vi "Process.vi"(8 "error in":errorcluster, 11 "Instrument.Example":refnum<class "Instrument.OxfordVRM.lvclass">) -> (0 "error out":errorcluster, 3 "Instrument.Example out":refnum<class "Instrument.OxfordVRM.lvclass">)   [LabVIEW 2016, in "Instrument.OxfordVRM.lvclass"]
doc: "---------------------------------------------------------------\nJKI State Machine Objects™\nhttp://jki.net/state-machine-objects/\nCopyright (C) 2005-2015, JKI <info@jki.net>\nALL RIGHTS RESERVED"
uses:
  Instrument.OxfordVRM.lvclass
  C:/Program Files (x86)/National Instruments/LabVIEW 2016/vi.lib/JKI/JKI SMO/SMO/SMO.lvclass
  <vilib>/JKI/JKI SMO/SMO/Typedefs/Parent Call--Enum.ctl
  <instrlib>/Mercury iXX/Public/Libraries/Magnet/Controls/Switch Heater.ctl
  <userlib>/LevyLab/Levylab Instruments/Instrument Types/Cryostat/Instrument.Cryostat.lvclass
  <vilib>/JKI/JKI SMO/SMO/SMO.lvclass
  <instrlib>/Mercury iXX/Public/Libraries/Magnet.lvlib
panel:
  out "State":string
  out "timer":u32
  # "For instructions on how to use the JKI State Machine Objects, examples and video tutorials, visit:\nhttp://jki.net/state-machine-objects/\n\nJKI State Machine Objects™\nhttp://jki.net/state-machine-objects/\nCopyright (C) 2005-2015, JKI <info@jki.net>\nALL RIGHTS RESERVED"
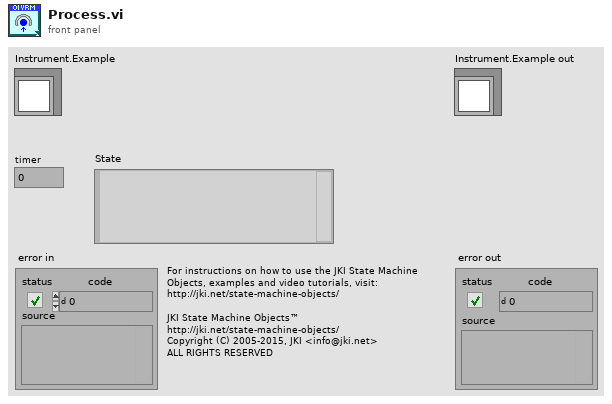
[diagram p1: front panel]
types:
  T1 = typedef "SMO.lvclass/Parent Call--Enum.ctl" = enum16{"Allows parent to run", "Does not request parent to run"}
  T2 = enum32{"invalid app kind", "Development System", "Run Time System", "Student Edition", "Embedded LabVIEW", "Evaluation", "Custom"}
  T3 = enum32{"Invalid", "Standard", "Closed", "Hidden", "Minimized", "Maximized"}
  T4 = enum32{"Bad", "Idle", "Run top level", "Running"}
  T5 = typedef "Mercury iXX.lvlib/Magnet.lvlib/Switch Heater.ctl" = string
  T6 = cluster{"Core":cluster{"Current VI Reference":refnum<vi>, "Close Panel on Exit?":bool, "error":errorcluster}, "Self Reference":refnum<class "Instrument.OxfordVRM.lvclass">, "Field (T)":dbl, "Field Rate (T/min)":dbl, "persistent":bool, "Running Step":i32, "sequence":string[]}
  T7 = cluster{"Current VI Reference":refnum<vi>, "Close Panel on Exit?":bool, "error":errorcluster}
  T8 = typedef "SMO.lvclass/Protected Events.ctl" = cluster{"StopProcesses":refnum<user-event>, "AbortProcesses":refnum<user-event>, "Config Changed":refnum<user-event>, "Dependency":refnum<user-event>}
  T9 = typedef "Instrument.OxfordVRM.lvclass/PrivateEvents--Cluster.ctl" = cluster{"SequenceSetMagnetField":refnum<user-event>, "AbortSequence":refnum<user-event>}
  T10 = cluster{"Holding":bool, "Ramp to Setpoint":bool, "Ramp to Zero":bool, "Clamp":bool}
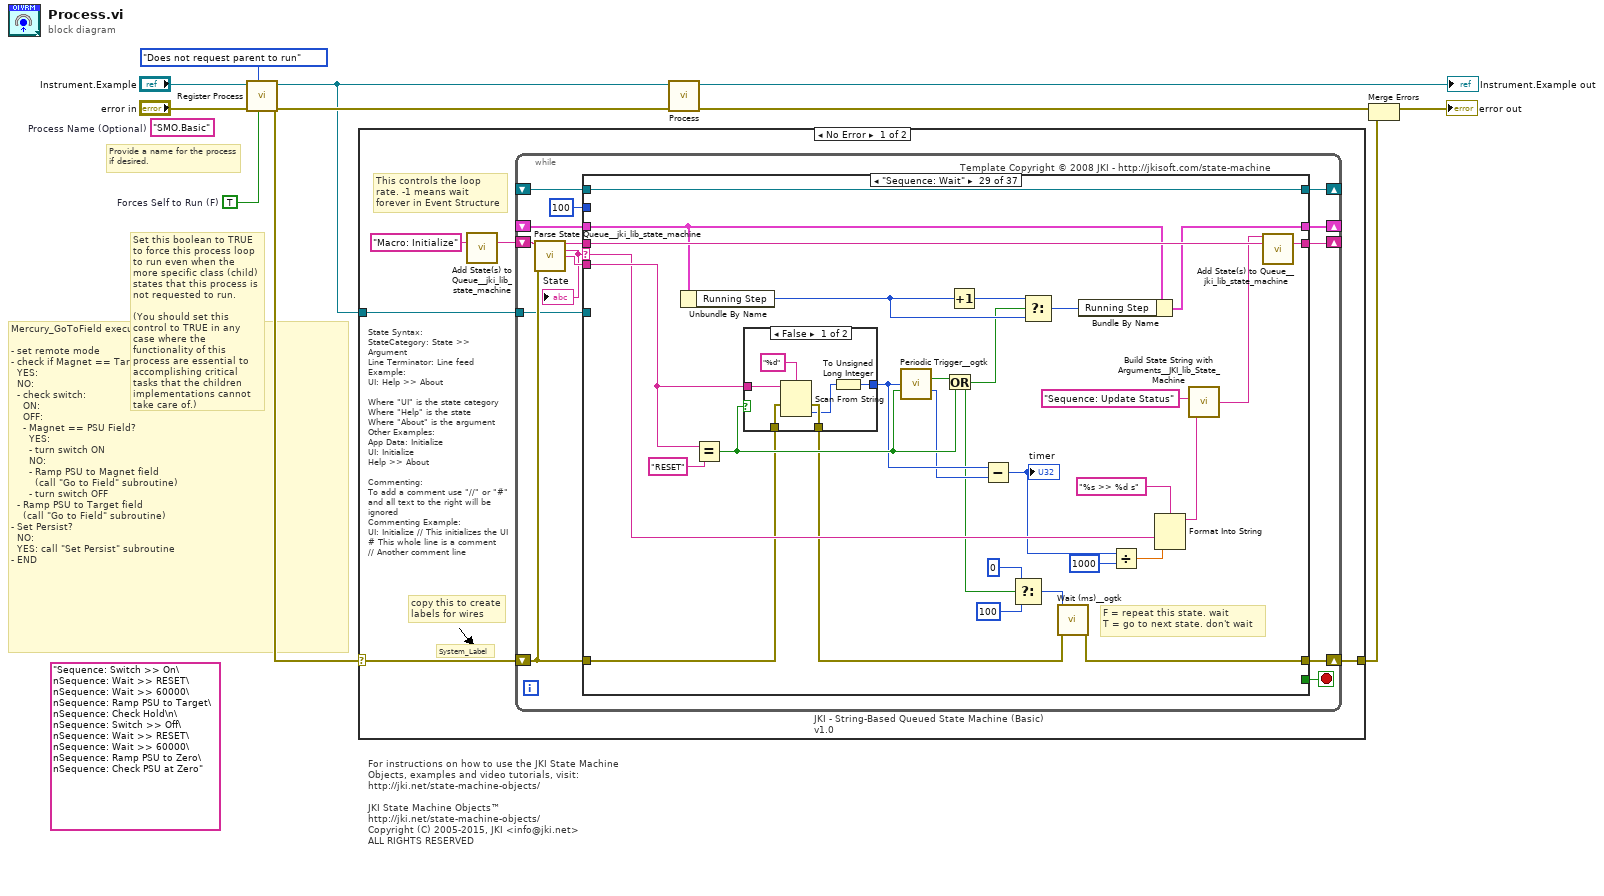
[diagram p0: block diagram]
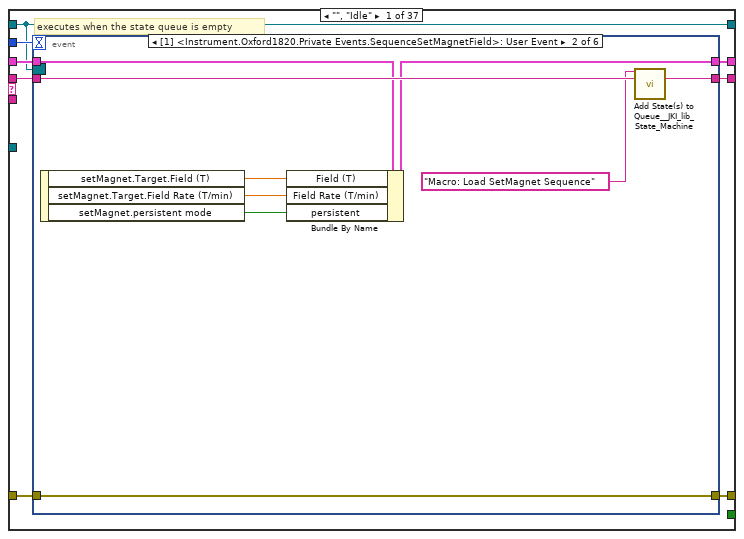
[diagram p2: hidden frame]
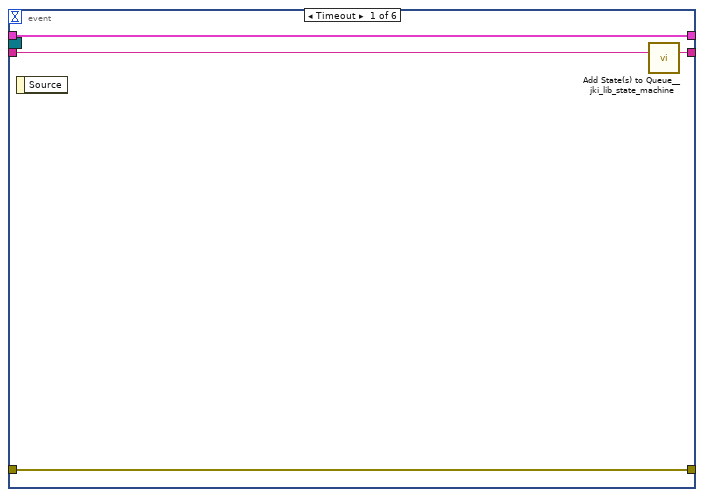
[diagram p3: hidden frame]
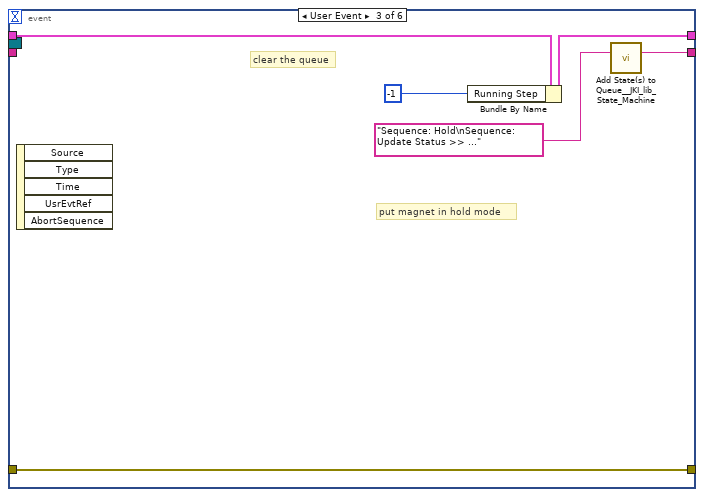
[diagram p4: hidden frame]
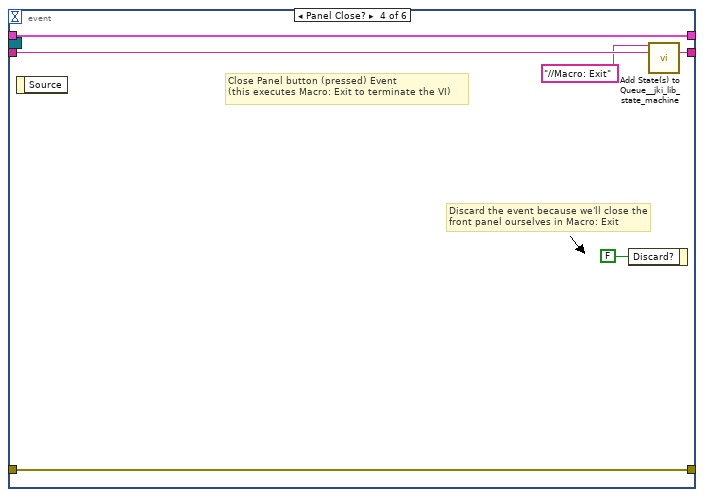
[diagram p5: hidden frame]
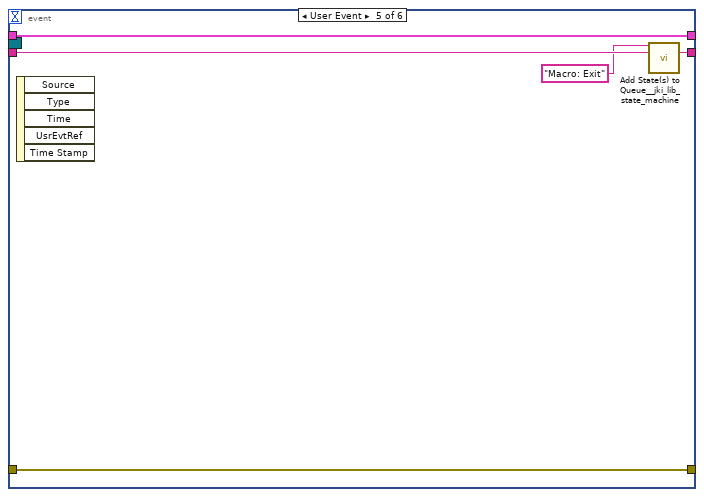
[diagram p6: hidden frame]
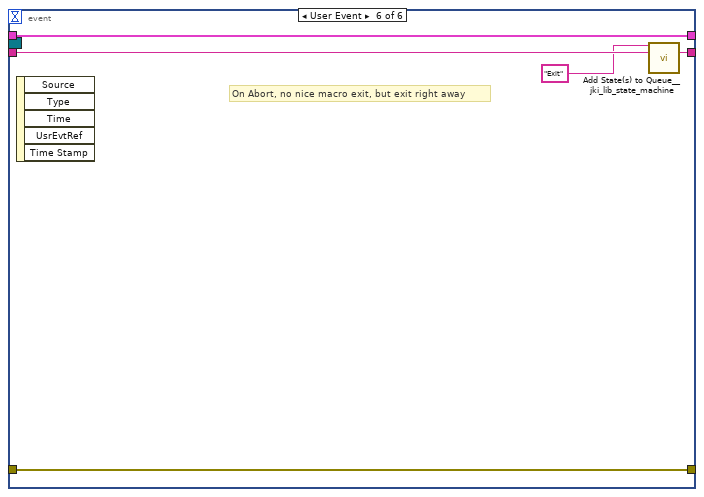
[diagram p7: hidden frame]
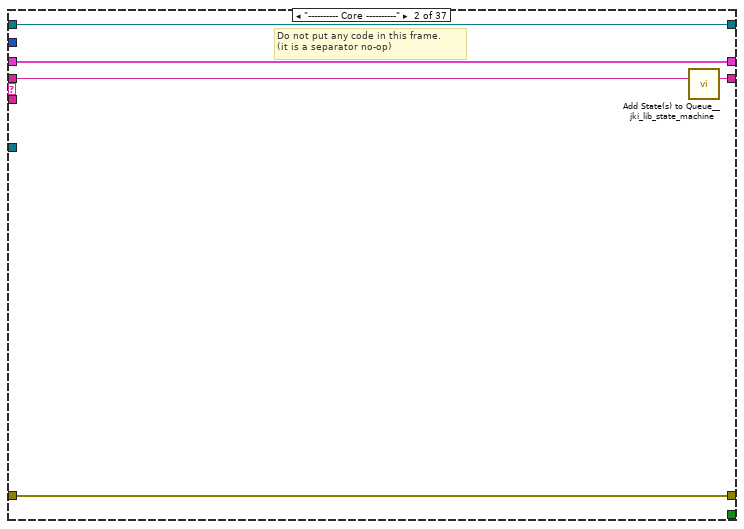
[diagram p8: hidden frame]
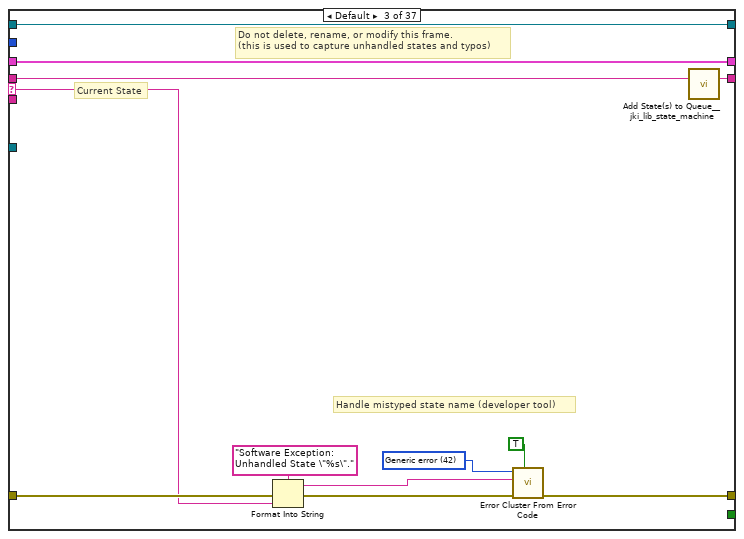
[diagram p9: hidden frame]
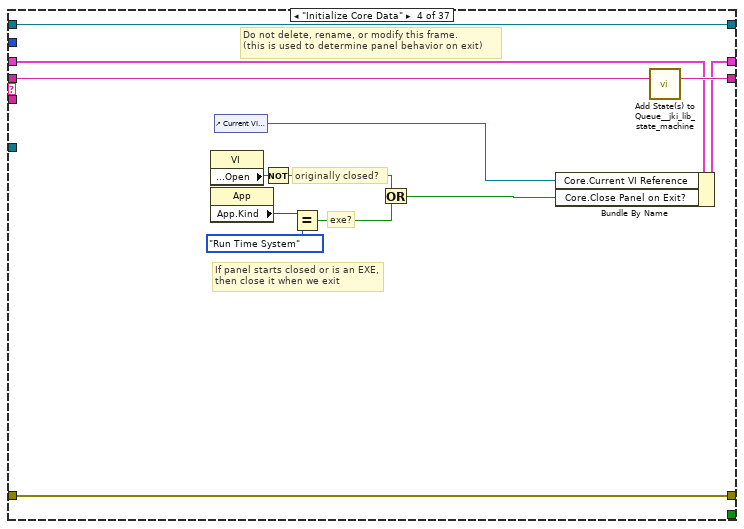
[diagram p10: hidden frame]
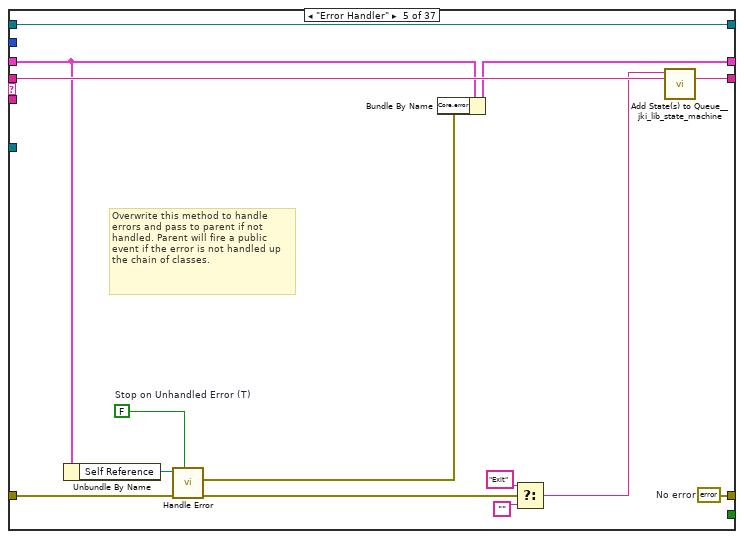
[diagram p11: hidden frame]
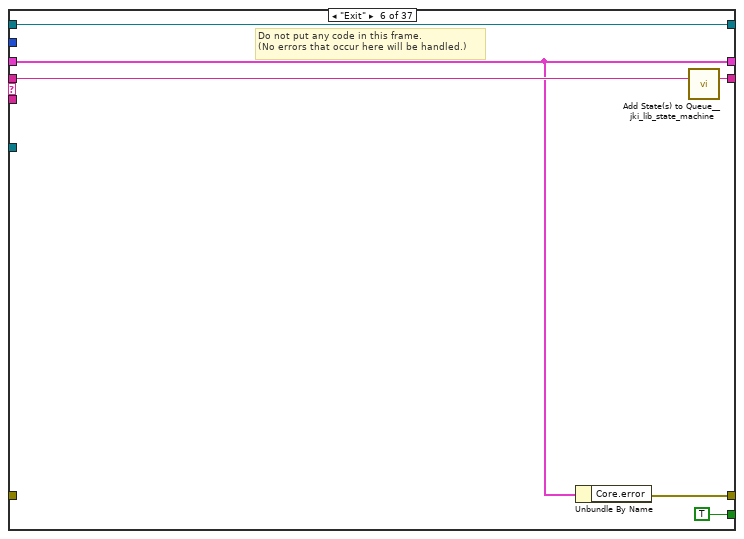
[diagram p12: hidden frame]
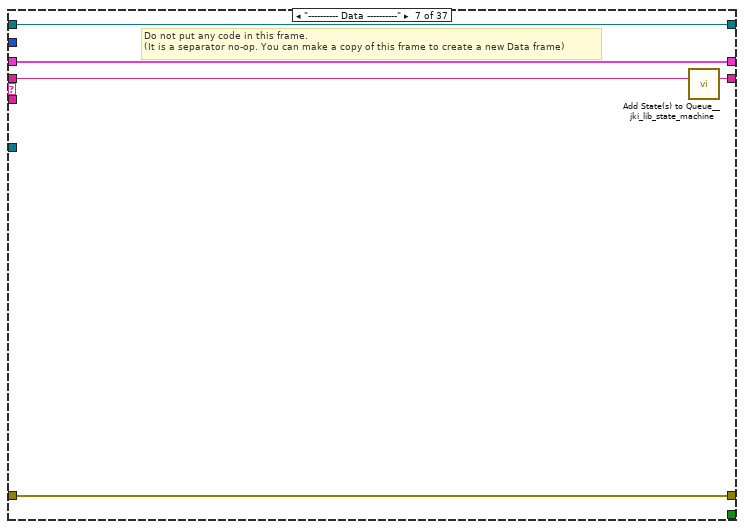
[diagram p13: hidden frame]
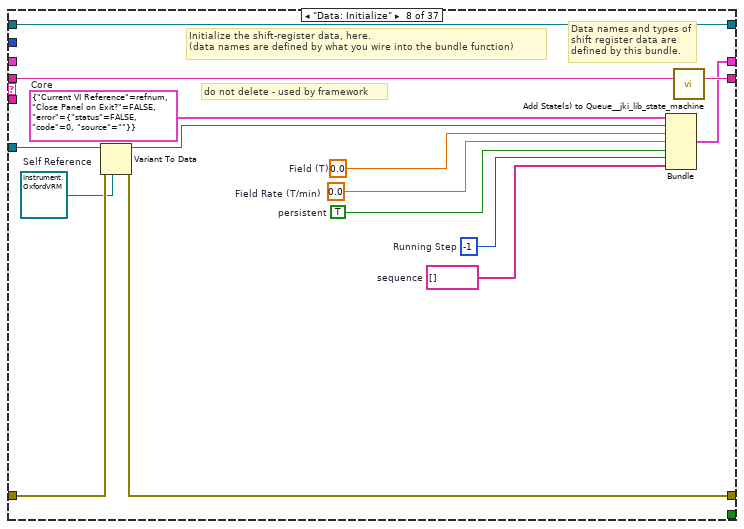
[diagram p14: hidden frame]
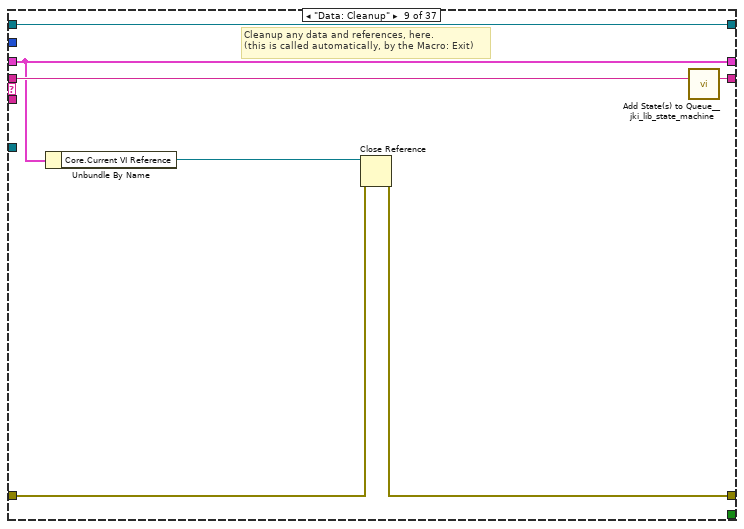
[diagram p15: hidden frame]
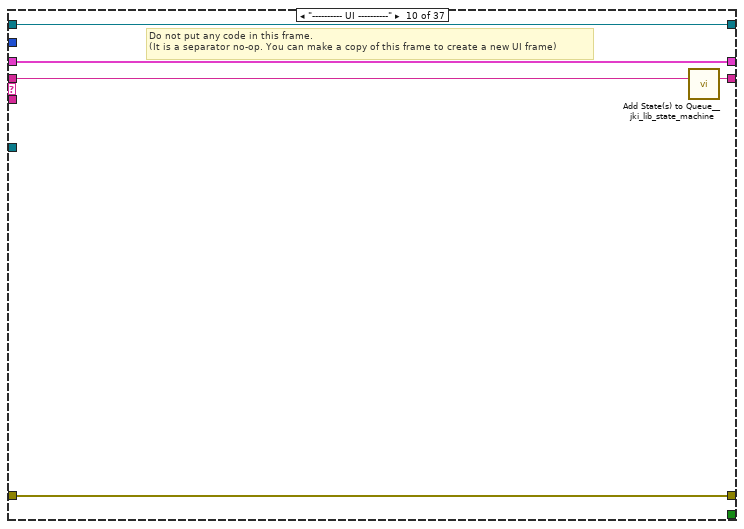
[diagram p16: hidden frame]
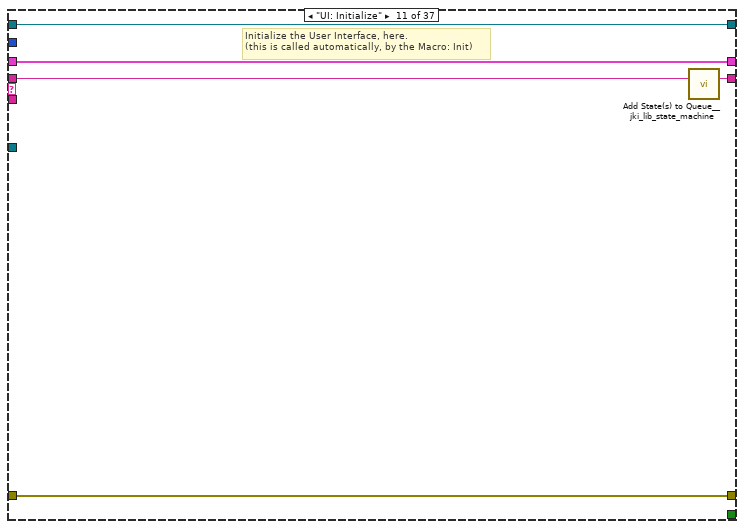
[diagram p17: hidden frame]
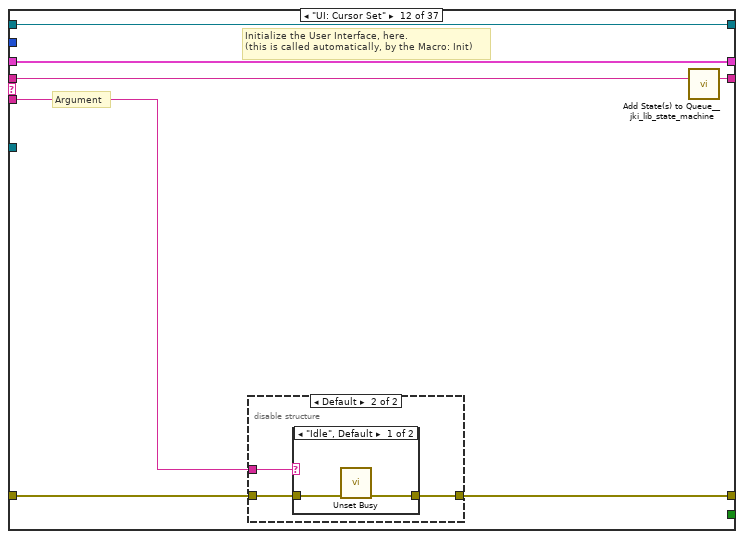
[diagram p18: hidden frame]
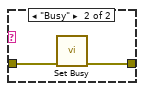
[diagram p20: hidden frame]
diagram:
  (unwired) "Sequence: Switch >> On\nSequence: Wait >> RESET\nSequence: Wait >> 60000\nSequence: Ramp PSU to Target\nSequence: Check Hold\n\nSequence: Switch >> Off\nSequence: Wait >> RESET\nSequence: Wait >> 60000\nSequence: Ramp PSU to Zero\nSequence: Check PSU at Zero" ("State(s) in Front (\"\")")
  w1 = TRUE  # Forces Self to Run (F)
  (unwired) "SMO.Basic"  # Process Name (Optional)
  # "Mercury_GoToField executes the following states:\n\n- set remote mode\n- check if Magnet == Target.\n  YES:\n  NO:\n  - check switch:\n    ON:\n    OFF:\n    - Magnet == PSU Field?\n      YES:\n      - turn switch ON\n      NO:\n      - Ramp PSU to Magnet field\n        (call \"Go to Field\" subroutine)\n      - turn switch OFF\n  - Ramp PSU to Target field\n    (call \"Go to Field\" subroutine)\n- Set Persist?\n  NO:\n  YES: call \"Set Persist\" subroutine\n- END"
  # "Provide a name for the process\nif desired."
  # "Set this boolean to TRUE to force this process loop to run even when the more specific class (child) states that this process is not requested to run.\n\n(You should set this control to TRUE in any case where the functionality of this process are essential to accomplishing critical tasks that the children implementations cannot take care of.)"
  # "For instructions on how to use the JKI State Machine Objects, examples and video tutorials, visit:\nhttp://jki.net/state-machine-objects/\n\nJKI State Machine Objects™\nhttp://jki.net/state-machine-objects/\nCopyright (C) 2005-2015, JKI <info@jki.net>\nALL RIGHTS RESERVED"
  n1 = call <vilib>:"Register Process.vi"("Forces Self to Run (F)"=w1, "Parent Call"=Parent_Call--Enum."Does not request parent to run", "error in (no error)"="error in", "SMO"="Instrument.Example") -> ("error out"=w7:errorcluster, "SMO out"=w6:refnum<class "Instrument.OxfordVRM.lvclass">)  [unwired: 6 in]
  n2 = case shown="No Error" w7 {
    selector: w7 -> [w12 w608]
    tunnel: w6 -> [w13 _]
    tunnel: [w11 w608] -> w3
    frame No Error {
      # "State Syntax:\nStateCategory: State >> Argument\nLine Terminator: Line feed\nExample:\nUI: Help >> About\n\nWhere \"UI\" is the state category\nWhere \"Help\" is the state\nWhere \"About\" is the argument\nOther Examples:\nApp Data: Initialize\nUI: Initialize\nHelp >> About\n\nCommenting:\nTo add a comment use \"//\" or \"#\" and all text to the right will be ignored\nCommenting Example:\nUI: Initialize // This initializes the UI\n# This whole line is a comment\n// Another comment line"
      # "copy this to create labels for wires"
      # "This controls the loop rate. -1 means wait forever in Event Structure"
      # "System_Label"
      n3 = call <vilib>:"Add State(s) to Queue__jki_lib_state_machine.vi"("State(s) in (\"\")"="Macro: Initialize") -> ("States Out"=w15:string)  [unwired: 14 in]
      n4 = while "JKI - String-Based Queued State Machine (Basic) v1.0" {
        shift-right: [w23] -> _
        shift-left: _ -> [w22]
        shift-right: [w26] -> w11
        shift-left: w12 -> [w20]
        shift-right: [w25] -> _
        shift-left: w15 -> [w27]
        tunnel: w13 -> [w19]
        shift-right: [w18] -> _
        shift-left: _ -> [w17]
        stop <- w24 stop-if-true
        # "Template Copyright © 2008 JKI - http://jkisoft.com/state-machine"
        n5 = call <vilib>:"Parse State Queue__jki_lib_state_machine.vi"("State Queue"=w27, "Error In (no error)"=w20) -> ("Remaining States"=w29:string, "Current State"=w16:string, "Arguments"=w28:string)  [unwired: 11 in]
        "State" <- w16
        n6 = case shown="\"Sequence: Wait\"" w16 {
          selector: w16 -> [_ _ w79 _ _ _ _ _ _ _ _ _ _ _ _ _ _ _ _ _ _ _ _ _ _ _ w363 w379 w407 w431 w460 w492 w509 w529 w549 w568 w598]
          tunnel: w29 -> [w37 w77 w83 w102 w116 w122 w127 w142 w149 w154 w159 w166 w182 w214 w235 w249 w266 _ w297 w308 w313 w326 w332 w341 w348 w358 w372 w389 w420 w447 w477 w500 w519 w539 w559 w580 w607]
          tunnel: w28 -> [_ _ _ _ _ _ _ _ _ _ _ w160 w176 _ _ _ _ _ _ _ _ _ _ _ _ w350 _ w378 w408 _ _ _ _ _ _ _ _]
          tunnel: w22 -> [w35 w74 w81 w93 w110 w118 w124 _ w144 w151 w157 w164 w178 w211 w232 w240 w254 w274 w294 w305 w310 w324 w330 w335 w344 w355 w369 w384 w393 w440 w473 w497 w512 w532 w552 w577 w604]
          tunnel: [w34 w75 w85 w99 w111 w117 w125 w138 w145 w152 w156 w161 w179 w212 w221 w247 w264 w270 w295 w299 w311 w319 w328 w338 w345 w351 w366 w381 w397 w434 w469 w488 w501 w521 w541 w560 w597] -> w26
          tunnel: w20 -> [w33 w75 w84 w99 w112 _ w125 w139 w146 w152 w156 w162 w180 w212 w222 w247 w264 w271 w295 w300 w311 w320 w328 w338 w345 w352 w361 w374 w396 w429 w458 w489 _ w520 w540 w562 w592]
          tunnel: [w36 w76 w82 w101 w115 w121 w126 w141 w148 w153 w158 w165 w181 w213 w234 w248 w265 w285 w296 w307 w312 w325 w331 w340 w347 w357 w371 w388 w419 w446 w476 w499 w518 w538 w558 w579 w606] -> w25
          tunnel: [_ _ _ _ _ TRUE _ _ _ _ _ _ _ _ _ _ _ _ _ _ _ _ _ _ _ _ _ _ _ _ _ _ _ _ _ _ _] -> w24
          tunnel: [w32 w74 w81 w100 w109 w118 w124 w140 w144 w151 w157 w164 w178 w211 w232 w240 w262 w275 w294 w305 w310 w324 w330 w334 w343 w354 w368 w383 w417 w439 w472 w496 w511 w531 w551 w576 w603] -> w23
          tunnel: 100 ("Timeout") -> [w31 _ _ _ _ _ _ _ _ _ _ _ _ _ _ _ _ _ _ _ _ _ _ _ _ _ _ _ _ _ _ _ _ _ _ _ _]
          tunnel: w19 -> [_ _ _ _ _ _ _ w136 _ _ _ _ _ _ w223 _ _ _ _ _ _ _ _ _ _ _ _ _ _ _ _ _ _ _ _ _ _]
          tunnel: [w30 w73 w78 w90 w114 w119 w123 w134 w143 w150 w155 w163 w175 w210 w233 w241 w263 w284 w293 w306 w309 w323 w329 w339 w346 w356 w370 w387 w418 w445 w475 w498 w517 w537 w557 w578 w605] -> w18
          tunnel: w17 -> [w30 w73 w78 w90 w114 w119 w123 w134 w143 w150 w155 w163 w175 w210 w233 w241 w263 w284 w293 w306 w309 _ w329 w339 w346 w356 w370 w387 w418 w445 w475 w498 w517 w537 w557 w578 w605]
          frame "", "Idle" {
            # "executes when the state queue is empty"
            n7 = event shown="[1] <Instrument.Oxford1820.Private Events.SequenceSetMagnetField>: User Event" {
              selector: w30 -> [_ _ _ _ _ _]
              dyn-events: _ -> [_ _ _ _ _ _]
              timeout: w31 -> [_ _ _ _ _ _]
              tunnel: w37 -> [w41 w48 _ w62 w67 w72]
              tunnel: [w40 w49 w55 w61 w66 w71] -> w36
              tunnel: w35 -> [w38 w44 w53 w59 w64 w69]
              tunnel: [w39 w50 w56 w60 w65 w70] -> w34
              tunnel: w33 -> [w39 w50 w56 w60 w65 w70]
              tunnel: [w38 w43 w52 w59 w64 w69] -> w32
              event Timeout {
                n8 = event-data() -> ()  [unwired: 1 in, 1 out]
                n9 = call <vilib>:"Add State(s) to Queue__jki_lib_state_machine.vi"("State(s) in (\"\")"=w41) -> ("States Out"=w40:string)  [unwired: 14 in]
              }
              event User Event {
                n10 = event-data() -> ("setMagnet.Target.Field (T)"=w47:dbl, "setMagnet.Target.Field Rate (T/min)"=w46:dbl, "setMagnet.persistent mode"=w45:bool)  [unwired: 1 in]
                n11 = Bundle By Name(cluster=w44, "Field (T)"=w47, "Field Rate (T/min)"=w46, "persistent"=w45) -> (w43:T6)
                n12 = call <vilib>:"Add State(s) to Queue__JKI_lib_State_Machine.vi"("State(s) in Front (\"\")"="Macro: Load SetMagnet Sequence" ("State(s) at Back (\"\")"), "State(s) in (\"\")"=w48) -> ("States Out"=w49:string)  [unwired: 13 in]
              }
              event User Event {
                # "put magnet in hold mode"
                # "clear the queue"
                n13 = event-data() -> ()  [unwired: 1 in, 5 out]
                n14 = Bundle By Name(cluster=w53, "Running Step"=-1) -> (w52:T6)
                n15 = call <vilib>:"Add State(s) to Queue__JKI_lib_State_Machine.vi"("State(s) in (\"\")"="Sequence: Hold\nSequence: Update Status >> ..." ("State(s) at Back (\"\")")) -> ("States Out"=w55:string)  [unwired: 14 in]
              }
              event Panel Close? {
                # "Discard the event because we'll close the front panel ourselves in Macro: Exit"
                # "Close Panel button (pressed) Event\n(this executes Macro: Exit to terminate the VI)"
                n16 = event-data() -> ()  [unwired: 1 in, 1 out]
                n17 = event-data("Discard?"=FALSE) -> ()  [unwired: 1 in, 1 out]
                n18 = call <vilib>:"Add State(s) to Queue__jki_lib_state_machine.vi"("State(s) in Front (\"\")"="//Macro: Exit", "State(s) in (\"\")"=w62) -> ("States Out"=w61:string)  [unwired: 13 in]
              }
              event User Event {
                n19 = event-data() -> ()  [unwired: 1 in, 5 out]
                n20 = call <vilib>:"Add State(s) to Queue__jki_lib_state_machine.vi"("State(s) in Front (\"\")"="Macro: Exit", "State(s) in (\"\")"=w67) -> ("States Out"=w66:string)  [unwired: 13 in]
              }
              event User Event {
                # "On Abort, no nice macro exit, but exit right away"
                n21 = event-data() -> ()  [unwired: 1 in, 5 out]
                n22 = call <vilib>:"Add State(s) to Queue__jki_lib_state_machine.vi"("State(s) in Front (\"\")"="Exit", "State(s) in (\"\")"=w72) -> ("States Out"=w71:string)  [unwired: 13 in]
              }
            }
          }
          frame "---------- Core ----------" {
            # "Do not put any code in this frame.\n(it is a separator no-op)"
            n23 = call <vilib>:"Add State(s) to Queue__jki_lib_state_machine.vi"("State(s) in (\"\")"=w77) -> ("States Out"=w76:string)  [unwired: 14 in]
          }
          frame Default {
            w88 = 42 items=["No error", "Argument error", "Memory is full", "Out of zone", "End of file", "File already open", "Generic file I/O error", "File not found", "File permission error", "Disk is full", "Duplicate path", "Too many files open", "System feature not enabled", "Resource file not found", "Cannot add resource", "Resource not found", "Image not found", "Image memory error", "Pen does not exist", "Config type invalid", "Config token not found", "Config parse error", "Config memory error", "Bad external code format", "Bad external code offset", "External code not present", "Null window", "Destroy window error", "Null menu", "Print aborted", "Bad print record", "Print driver error", "Windows error during printing", "Memory error during printing", "Print dialog error", "Generic print error", "Invalid device refnum", "Device not found", "Device parameter error", "Device unit error", "Cannot open device", "Device call aborted", "Generic error", "Cancelled by user", "Object ID too low", "Object ID too high", "Object not in heap", "Unknown heap", "Unknown object (invalid DefProc)", "Unknown object (DefProc not in table)", "Message out of range", "Invalid (null) method", "Unknown message", "Manager call not supported", "Bad address", "Network operation in progress", "Network operation timed out", "Connection is busy", "Network attribute not supported", "Network error", "Address in use", "System out of memory", "Connection aborted", "Connection refused", "Not connected", "Already connected", "Connection closed", "Initialization error (interapplication manager)", "Bad occurrence", "Wait on unbound occurrence handler", "Occurrence queue overflow", "Datalog type conflict", "Unused", "Unrecognized type (interapplication manager)", "Memory corrupt", "Failed to make temporary DLL", "Old CIN version", "Drag socket not found", "Failed to load drop-object", "Failed to register OLE object", "Failed to release OLE object", "Format specifier type mismatch", "Unknown format specifier", "Too few format specifiers", "Too many format specifiers", "Scan failed", "Newer CIN version", "Error converting to variant", "Runtime menu error", "Password tampered", "Variant attribute not found", "Incompatible variant data type", "Event data is not available", "Event Store is not present", "Occurrence is not found", "Event Queue is not created", "Event info is not available", "Refnum passed is NULL", "Error retrieving Class GUID", "Error retrieving CoClass GUID", "Error retrieving TypeLib GUID.", "Bad built application magic bytes.", "Specific driver is different from the specific driver associated with the Logical Name.", "There is no session opened to the class driver.", "Max Error", "MAX - Error with config objects", "MAX - Error loading configuration", "MAX - Group not supported"]
            # "Current State"
            # "Do not delete, rename, or modify this frame.\n(this is used to capture unhandled states and typos)"
            # "Handle mistyped state name (developer tool)"
            n24 = Format Into String(format string="Software Exception: Unhandled State \"%s\"." ("message"), error in=w84, w79) -> (resulting string=w87:string, error out=w86:errorcluster)  [unwired: 1 in]
            n25 = call <vilib>:"Error Cluster From Error Code.vi"("show call chain? (False)"=TRUE, "error in (no error)"=w86, "error message (\"\")"=w87, "error code (0)"=w88) -> ("error out"=w85:errorcluster)  [unwired: 5 in]
            n26 = call <vilib>:"Add State(s) to Queue__jki_lib_state_machine.vi"("State(s) in (\"\")"=w83) -> ("States Out"=w82:string)  [unwired: 14 in]
          }
          frame "Initialize Core Data" {
            # "Do not delete, rename, or modify this frame.\n(this is used to determine panel behavior on exit)"
            # "originally closed?"
            # "exe?"
            # "If panel starts closed or is an EXE, then close it when we exit"
            n27 = property class="VI"() -> ("Front Panel.Open"=w98:bool)  [unwired: 2 in, 2 out]
            n28 = property class="App"() -> ("App.Kind"=w97:T2)  [unwired: 2 in, 2 out]
            n29 = control-ref of="Current VI Reference"() -> (w91:refnum<vi>)
            n30 = Not(x=w98) -> (.not. x?=w95:bool)
            n31 = Equal?(x=w97, y=T2."Run Time System" ("Application:Kind")) -> (x = y?=w94:bool)
            n32 = Or(x=w95, y=w94) -> (x .or. y?=w92:bool)
            n33 = Bundle By Name(cluster=w93, "Core.Current VI Reference"=w91, "Core.Close Panel on Exit?"=w92) -> (w100:T6)
            n34 = call <vilib>:"Add State(s) to Queue__jki_lib_state_machine.vi"("State(s) in (\"\")"=w102) -> ("States Out"=w101:string)  [unwired: 14 in]
          }
          frame "Error Handler" {
            w103 = FALSE  # Stop on Unhandled Error (T)
            w111 = errorcluster {"status"=FALSE, "code"=0, "source"=""}  # No error
            # "Overwrite this method to handle errors and pass to parent if not handled. Parent will fire a public event if the error is not handled up the chain of classes."
            n35 = Unbundle By Name(w110) -> ("Self Reference"=w113:refnum<class "Instrument.OxfordVRM.lvclass">)
            n36 = call-dynamic "Handle Error.vi"("Stop on Unhandled Error (T)"=w103, "error in"=w112, "Instrument"=w113) -> ("handling error"=w104:errorcluster, "Unhandled error"=w107:errorcluster)  [unwired: 6 in, 1 out]
            n37 = Bundle By Name(cluster=w110, "Core.error"=w107) -> (w109:T6)
            n38 = Select(t="Exit", s=w104, f="") -> (s? t:f=w108:string)
            n39 = call <vilib>:"Add State(s) to Queue__jki_lib_state_machine.vi"("State(s) in Front (\"\")"=w108, "State(s) in (\"\")"=w116) -> ("States Out"=w115:string)  [unwired: 13 in]
          }
          frame "Exit" {
            # "Do not put any code in this frame.\n(No errors that occur here will be handled.)"
            n40 = Unbundle By Name(w118) -> ("Core.error"=w117:errorcluster)
            n41 = call <vilib>:"Add State(s) to Queue__jki_lib_state_machine.vi"("State(s) in (\"\")"=w122) -> ("States Out"=w121:string)  [unwired: 14 in]
          }
          frame "---------- Data ----------" {
            # "Do not put any code in this frame.\n(It is a separator no-op. You can make a copy of this frame to create a new Data frame)"
            n42 = call <vilib>:"Add State(s) to Queue__jki_lib_state_machine.vi"("State(s) in (\"\")"=w127) -> ("States Out"=w126:string)  [unwired: 14 in]
          }
          frame "Data: Initialize" {
            w128 = string[] []  # sequence
            w129 = -1  # Running Step
            w130 = TRUE  # persistent
            w131 = 0.0  # Field Rate (T/min)
            w132 = 0.0  # Field (T)
            w133 = T7 {"Current VI Reference"=refnum, "Close Panel on Exit?"=FALSE, "error"={"status"=FALSE, "code"=0, "source"=""}}  # Core
            w137 = refnum<class "Instrument.OxfordVRM.lvclass"> refnum  # Self Reference
            # "do not delete - used by framework"
            # "Data names and types of shift register data are defined by this bundle."
            # "Initialize the shift-register data, here.\n(data names are defined by what you wire into the bundle function)"
            n43 = Variant To Data(error in=w139, type=w137, Variant=w136) -> (data=w135:refnum<class "Instrument.OxfordVRM.lvclass">, error out=w138:errorcluster)
            n44 = Bundle("Core"=w133, "Self Reference"=w135, "Field (T)"=w132, "Field Rate (T/min)"=w131, "persistent"=w130, "Running Step"=w129, "sequence"=w128) -> (w140:T6)  [unwired: 1 in]
            n45 = call <vilib>:"Add State(s) to Queue__jki_lib_state_machine.vi"("State(s) in (\"\")"=w142) -> ("States Out"=w141:string)  [unwired: 14 in]
          }
          frame "Data: Cleanup" {
            # "Cleanup any data and references, here.\n(this is called automatically, by the Macro: Exit)"
            n46 = Unbundle By Name(w144) -> ("Core.Current VI Reference"=w147:refnum<vi>)
            n47 = Close Reference(reference=w147, error in (no error)=w146) -> (error out=w145:errorcluster)
            n48 = call <vilib>:"Add State(s) to Queue__jki_lib_state_machine.vi"("State(s) in (\"\")"=w149) -> ("States Out"=w148:string)  [unwired: 14 in]
          }
          frame "---------- UI ----------" {
            # "Do not put any code in this frame.\n(It is a separator no-op. You can make a copy of this frame to create a new UI frame)"
            n49 = call <vilib>:"Add State(s) to Queue__jki_lib_state_machine.vi"("State(s) in (\"\")"=w154) -> ("States Out"=w153:string)  [unwired: 14 in]
          }
          frame "UI: Initialize" {
            # "Initialize the User Interface, here.\n(this is called automatically, by the Macro: Init)"
            n50 = call <vilib>:"Add State(s) to Queue__jki_lib_state_machine.vi"("State(s) in (\"\")"=w159) -> ("States Out"=w158:string)  [unwired: 14 in]
          }
          frame "UI: Cursor Set" {
            # "Argument"
            # "Initialize the User Interface, here.\n(this is called automatically, by the Macro: Init)"
            n51 = disable-structure shown="Default" {
              disable-tunnel: w162 -> [w167 w170]
              disable-tunnel: [w167 w169] -> w161
              disable-tunnel: w160 -> [_ w168]
              frame condition #0 {
              }
              frame condition #1 (active) {
                n52 = case shown="\"Idle\", Default" w168 {
                  tunnel: w170 -> [w172 w174]
                  tunnel: [w171 w173] -> w169
                  frame "Idle", Default {
                    n53 = call <vilib>:"Unset Busy.vi"("error in (no error)"=w172) -> ("error out"=w171:errorcluster)  [unwired: 10 in]
                  }
                  frame "Busy" {
                    n54 = call <vilib>:"Set Busy.vi"("error in (no error)"=w174) -> ("error out"=w173:errorcluster)  [unwired: 9 in, 1 out]
                  }
                }
              }
            }
            n55 = call <vilib>:"Add State(s) to Queue__jki_lib_state_machine.vi"("State(s) in (\"\")"=w166) -> ("States Out"=w165:string)  [unwired: 14 in]
          }
          frame "UI: Front Panel State" {
            # "Argument"
            # "Set Front Panel Open or Closed\n(Usage: \"UI: Front Panel State >> Open|Close\")"
            n56 = Unbundle By Name(w178) -> ("Core.Current VI Reference"=w177:refnum<vi>)
            n57 = disable-structure shown="Default" {
              disable-tunnel: w180 -> [w186 w209]
              disable-tunnel: [w185 w209] -> w179
              disable-tunnel: w177 -> [w184 _]
              disable-tunnel: w176 -> [w183 _]
              frame condition #0 (active) {
                n58 = case shown="\"Close\"" w183 {
                  tunnel: w186 -> [w190 w203]
                  tunnel: [w192 w204] -> w185
                  tunnel: w184 -> [w191 w201]
                  frame "Open", Default {
                    n59 = property class="VI"(reference=w191, error in=w190) -> (reference out=w188:refnum<vi>, error out=w189:errorcluster, "FP.State"=w187:T3)
                    n60 = case shown="\"Closed\"" w187 {
                      tunnel: [w195 w198] -> w192
                      tunnel: w189 -> [w194 w198]
                      tunnel: w188 -> [w193 _]
                      frame "Closed" {
                        n61 = invoke class="VI" method="FP.Open"(reference=w193, error in=w194, "Activate"=TRUE, "State"=T3."Standard") -> (error out=w195:errorcluster)  [unwired: 1 in, 4 out]
                      }
                      frame Default {
                      }
                    }
                  }
                  frame "Close" {
                    n62 = property class="VI"(reference=w201, error in=w203) -> (reference out=w200:refnum<vi>, error out=w202:errorcluster, "FP.State"=w199:T3)
                    n63 = case shown="Default" w199 {
                      tunnel: [w205 w208] -> w204
                      tunnel: w202 -> [w205 w207]
                      tunnel: w200 -> [_ w206]
                      frame "Invalid", "Closed" {
                      }
                      frame Default {
                        n64 = invoke class="VI" method="FP.Close"(reference=w206, error in=w207) -> (error out=w208:errorcluster)  [unwired: 1 in, 2 out]
                      }
                    }
                  }
                }
              }
              frame condition #1 {
              }
            }
            n65 = call <vilib>:"Add State(s) to Queue__jki_lib_state_machine.vi"("State(s) in (\"\")"=w182) -> ("States Out"=w181:string)  [unwired: 14 in]
          }
          frame "---------- Macro ----------" {
            # "Do not put any code in this frame.\n(It is a separator no-op. You can make a copy of this frame to create a new Macro frame)"
            n66 = call <vilib>:"Add State(s) to Queue__jki_lib_state_machine.vi"("State(s) in (\"\")"=w214) -> ("States Out"=w213:string)  [unwired: 14 in]
          }
          frame "Macro: Initialize" {
            w216 = "UI: Initialize\nUI: Front Panel State >> %s"  # UI: Initialize UI: Front Panel State >> %s
            w224 = "Process: Sync"
            # "Initialization Macro\n(This is called once, when the VI starts)"
            n67 = control-ref of="This VI"() -> (w226:refnum<vi>)
            n68 = property class="VI"(reference=w226) -> ("Exec.State"=w225:T4)  [unwired: 1 in, 2 out]
            n69 = call-dynamic "Read Debug Mode.vi"("error in (no error)"=w222, "Instrument in"=w223) -> ("error out"=w221:errorcluster, "Debug Mode?"=w218:bool)  [unwired: 7 in, 1 out]
            n70 = Equal?(x=w225, y=T4."Run top level") -> (x = y?=w230:bool)
            n71 = Select(t="Open", s=w218, f="Close") -> (s? t:f=w217:string)
            n72 = Select(t=w224, s=w230, f="") -> ()  [unwired: 1 out]
            n73 = Format Into String(format string=w216, w217) -> (resulting string=w215:string)  [unwired: 2 in, 1 out]
            n74 = call <vilib>:"Add State(s) to Queue__jki_lib_state_machine.vi"("State(s) in Front (\"\")"="Data: Initialize\nInitialize Core Data\nEvents: Register", "State(s) in (\"\")"=w224, "State(s) at Back (\"\")"=w215) -> ("States Out"=w227:string)  [unwired: 12 in]
            n75 = call <vilib>:"Add State(s) to Queue__jki_lib_state_machine.vi"("State(s) in Front (\"\")"=w227, "State(s) in (\"\")"=w235) -> ("States Out"=w234:string)  [unwired: 13 in]
          }
          frame "Macro: Exit" {
            # "Exit Macro\n(This is called once, when the VI exits)"
            n76 = Unbundle By Name(w240) -> ("Core.Close Panel on Exit?"=w246:bool)
            n77 = Select(t="UI: Front Panel State >> Close", s=w246, f="") -> (s? t:f=w243:string)
            n78 = call <vilib>:"Add State(s) to Queue__jki_lib_state_machine.vi"("State(s) in Front (\"\")"="Data: Cleanup\nEvents: Unregister", "State(s) in (\"\")"="Process: Sync", "State(s) at Back (\"\")"="Exit") -> ("States Out"=w237:string)  [unwired: 12 in]
            n79 = call <vilib>:"Add State(s) to Queue__jki_lib_state_machine.vi"("State(s) in (\"\")"=w243, "State(s) at Back (\"\")"=w237) -> ("States Out"=w242:string)  [unwired: 13 in]
            n80 = call <vilib>:"Add State(s) to Queue__jki_lib_state_machine.vi"("State(s) in Front (\"\")"=w242, "State(s) in (\"\")"=w249) -> ("States Out"=w248:string)  [unwired: 13 in]
          }
          frame "Macro: Run Sequence" {
            # "0,1,2,3,4,"
            # "5"
            # "Do not put any code in this frame.\n(It is a separator no-op. You can make a copy of this frame to create a new Macro frame)"
            n81 = Unbundle By Name(w254) -> ("sequence"=w260:string[], "Running Step"=w252:i32)
            n82 = Index Array(array=w260, index=w252) -> (element=w258:string)
            n83 = Array Size(array=w260) -> (size(s)=w261:i32)
            n84 = Equal?(x=w261, y=w252) -> (x = y?=w253:bool)
            n85 = Select(t=-1 ("Running Step"), s=w253, f=w252) -> (s? t:f=w259:i32)
            n86 = Select(t="Sequence: Update Status >> ...", s=w253, f="Idle\nMacro: Run Sequence" ("State(s) at Back (\"\")")) -> (s? t:f=w255:string)
            n87 = Bundle By Name(cluster=w254, "Running Step"=w259) -> (w262:T6)
            n88 = call <vilib>:"Add State(s) to Queue__jki_lib_state_machine.vi"("State(s) in Front (\"\")"=w258, "State(s) at Back (\"\")"=w255) -> ("States Out"=w257:string)  [unwired: 13 in]
            n89 = call <vilib>:"Add State(s) to Queue__jki_lib_state_machine.vi"("State(s) in Front (\"\")"=w257, "State(s) in (\"\")"=w266) -> ("States Out"=w265:string)  [unwired: 13 in]
          }
          frame "Macro: Load SetMagnet Sequence" {
            # "clear the queue"
            # "Do not put any code in this frame.\n(It is a separator no-op. You can make a copy of this frame to create a new Macro frame)"
            n90 = Unbundle By Name(w274) -> ("persistent"=w283:bool)
            n91 = Unbundle By Name(w274) -> ("Self Reference"=w273:refnum<class "Instrument.OxfordVRM.lvclass">, "Field (T)"=w269:dbl)
            n92 = call "Get Field.vi"("error in (no error)"=w271, "Instrument.1820 in"=w273) -> ("error out"=w270:errorcluster, "Field (T)"=w268:dbl)  [unwired: 7 in, 1 out]
            n93 = call "Instrument.1820.FloatApprox.vi"("y"=w269, "x"=w268) -> ("x ~ y?"=w272:bool)  [unwired: 4 in]
            n94 = Select(t="Sequence: Switch >> Off\nSequence: Wait >> RESET\nSequence: Wait >> 60000\nSequence: Ramp PSU to Zero\nSequence: Check Hold" ("State(s) in Front (\"\")"), s=w283, f="") -> (s? t:f=w281:string)
            n95 = call <vilib>:"Add State(s) to Queue__jki_lib_state_machine.vi"("State(s) in Front (\"\")"="Sequence: Hold\nSequence: Check Hold\nSequence: Ramp PSU to Magnet\nSequence: Check Hold\nSequence: Switch >> On\nSequence: Wait >> RESET\nSequence: Wait >> 60000\nSequence: Ramp PSU to Target\nSequence: Check Hold" ("State(s) in Front (\"\")"), "State(s) at Back (\"\")"=w281) -> ("States Out"=w267:string)  [unwired: 13 in]
            n96 = call <userlib>:"String to 1D Array__ogtk.vi"("delimiter (Tab)"="\n", "string"=w267) -> ("Array of Strings"=w279:string[])  [unwired: 9 in]
            n97 = case shown="False" w272 {
              tunnel: w279 -> [w289 _]
              tunnel: ["Macro: Run Sequence" ("State(s) in Front (\"\")") "" ("State(s) in Front (\"\")")] -> w277
              tunnel: [w287 w291] -> w275
              tunnel: w274 -> [w286 w291]
              frame False {
                n98 = Bundle By Name(cluster=w286, "Running Step"=0 ("sequence"), "sequence"=w289) -> (w287:T6)
              }
              frame True {
              }
            }
            n99 = call <vilib>:"Add State(s) to Queue__jki_lib_state_machine.vi"("State(s) in Front (\"\")"=w277) -> ("States Out"=w285:string)  [unwired: 14 in]
          }
          frame "---------- Process ----------" {
            # "Template Separator\n(You can make a copy of, or modify, this frame)"
            n100 = call <vilib>:"Add State(s) to Queue__jki_lib_state_machine.vi"("State(s) in (\"\")"=w297) -> ("States Out"=w296:string)  [unwired: 14 in]
          }
          frame "Process: Sync" {
            n101 = Unbundle By Name(w305) -> ("Self Reference"=w301:refnum<class "Instrument.OxfordVRM.lvclass">)
            n102 = call <vilib>:"WaitOnProcessSync.vi"("error in (no error)"=w300, "SMO"=w301) -> ("error out"=w299:errorcluster, "Don't run?"=w304:bool)  [unwired: 7 in, 1 out]
            n103 = Select(t="Data: Cleanup\nEvents: Unregister\nExit", s=w304, f="") -> (s? t:f=w298:string)
            n104 = call <vilib>:"Add State(s) to Queue__jki_lib_state_machine.vi"("State(s) in Front (\"\")"=w298, "State(s) in (\"\")"=w308) -> ("States Out"=w307:string)  [unwired: 13 in]
          }
          frame "---------- Events ----------" {
            # "Template Separator\n(You can make a copy of, or modify, this frame)"
            n105 = call <vilib>:"Add State(s) to Queue__jki_lib_state_machine.vi"("State(s) in (\"\")"=w313) -> ("States Out"=w312:string)  [unwired: 14 in]
          }
          frame "Events: Register" {
            # "Expand to add\nmore events"
            n106 = Unbundle By Name(w324) -> ("Self Reference"=w321:refnum<class "Instrument.OxfordVRM.lvclass">)
            n107 = call <vilib>:"GetProtectedEvents.vi"("SMO"=w321) -> ("error out"=w317:errorcluster, "SMO Protected Events"=w322:T8, "SMO out"=w316:refnum<class "Instrument.OxfordVRM.lvclass">)  [unwired: 8 in]
            n108 = call "Instrument.Oxford1820.GetPrivateEvents.vi"("Instrument.Oxford1820"=w316) -> ("error out"=w315:errorcluster, "Instrument.Oxford1820.Private Events"=w314:T9)  [unwired: 8 in, 1 out]
            n109 = register-events(w322, w314) -> (reference out=w323:refnum<event-registration>, error out=w318:errorcluster)  [unwired: 2 in]
            n110 = Merge Errors(w315, w320, w318, w317) -> (w319:errorcluster)
            n111 = call <vilib>:"Add State(s) to Queue__jki_lib_state_machine.vi"("State(s) in (\"\")"=w326) -> ("States Out"=w325:string)  [unwired: 14 in]
          }
          frame "Events: Unregister" {
            n112 = Unregister For Events(event registration refnum=w329, error in=w328) -> (error out=w327:errorcluster)
            n113 = call <vilib>:"Clear Errors.vi"("error in (no error)"=w327) -> ()  [unwired: 5 in, 2 out]
            n114 = call <vilib>:"Add State(s) to Queue__jki_lib_state_machine.vi"("State(s) in (\"\")"=w332) -> ("States Out"=w331:string)  [unwired: 14 in]
          }
          frame "---------- Sequence ----------" {
            n115 = Unbundle By Name(w335) -> ("Running Step"=w333:i32, "Self Reference"=w337:refnum<class "Instrument.OxfordVRM.lvclass">)
            n116 = Increment(x=w333) -> (x+1=w336:i32)
            n117 = Bundle By Name(cluster=w335, "Running Step"=w336, "Self Reference"=w337) -> (w334:T6)
            n118 = call <vilib>:"Add State(s) to Queue__jki_lib_state_machine.vi"("State(s) in (\"\")"=w341) -> ("States Out"=w340:string)  [unwired: 14 in]
          }
          frame "Sequence: Template" {
            # "switch ON/OFF:\n- include checks for PSU == Magnet.\n- call \"Go to Field\" as needed to make PSU == Magnet"
            # "\"Set Persist\" subroutine:\n\n- switch on?\n  NO:\n  YES:\n  - turn switch OFF\n- Ramp PSU to 0\n  (call \"Go to Field\" subroutine)\n- END"
            # "\"Go to Field\" subroutine:\n\n- set to remote mode (obsolete?)\n- write target field.\n  check and resend if necessary\n- put in hold mode.\n  check and resend if necessary\n- check if Target = PSU:\n  YES:\n  NO:\n  - put in GTOS mode. check and resend if necessary\n- wait until PSU is in hold mode\n  (PSU will go to hold mode once PSU @ target)\n- END"
            # "Mercury_GoToField executes the following states:\n\n- set remote mode (obsolete?)\n- check if Magnet == Target.\n  YES:\n  NO:\n  - check switch:\n    ON:\n    OFF:\n    - Magnet == PSU Field?\n      YES:\n      - turn switch ON\n      NO:\n      - Ramp PSU to Magnet field\n        (call \"Go to Field\" subroutine)\n      - turn switch OFF\n  - Ramp PSU to Target field\n    (call \"Go to Field\" subroutine)\n- Set Persist?\n  NO:\n  YES: call \"Set Persist\" subroutine\n- END"
            n119 = Unbundle By Name(w344) -> ("Self Reference"=w342:refnum<class "Instrument.OxfordVRM.lvclass">)
            n120 = Bundle By Name(cluster=w344, "Self Reference"=w342) -> (w343:T6)
            n121 = call <vilib>:"Add State(s) to Queue__jki_lib_state_machine.vi"("State(s) in (\"\")"=w348) -> ("States Out"=w347:string)  [unwired: 14 in]
          }
          frame "Sequence: Update Status" {
            n122 = Unbundle By Name(w355) -> ("Self Reference"=w353:refnum<class "Instrument.OxfordVRM.lvclass">)
            n123 = call "Instrument.Oxford1820.ProcessStatus.vi"("error in (no error)"=w352, "event data"=w350, "Instrument.Oxford1820"=w353) -> ("error out"=w351:errorcluster, "Instrument.Oxford1820 out"=w349:refnum<class "Instrument.OxfordVRM.lvclass">)  [unwired: 7 in]
            n124 = Bundle By Name(cluster=w355, "Self Reference"=w349) -> (w354:T6)
            n125 = call <vilib>:"Add State(s) to Queue__jki_lib_state_machine.vi"("State(s) in (\"\")"=w358) -> ("States Out"=w357:string)  [unwired: 14 in]
          }
          frame "Sequence: Hold" {
            n126 = Unbundle By Name(w369) -> ("Running Step"=w360:i32, "Self Reference"=w362:refnum<class "Instrument.OxfordVRM.lvclass">)
            n127 = Increment(x=w360) -> (x+1=w359:i32)
            n128 = call "Hold.vi"("error in (no error)"=w361, "Instrument.1820 in"=w362) -> ("error out"=w366:errorcluster, "Instrument.1820 in"=w367:refnum<class "Instrument.OxfordVRM.lvclass">)  [unwired: 7 in, 1 out]
            n129 = Bundle By Name(cluster=w369, "Running Step"=w359, "Self Reference"=w367) -> (w368:T6)
            n130 = call <vilib>:"Build State String with Arguments__JKI_lib_State_Machine.vi"("Arguments (\"\")"=w363, "State"="Sequence: Update Status") -> ("State with Arguments"=w365:string)  [unwired: 4 in]
            n131 = call <vilib>:"Add State(s) to Queue__jki_lib_state_machine.vi"("State(s) in Front (\"\")"=w365, "State(s) in (\"\")"=w372) -> ("States Out"=w371:string)  [unwired: 13 in]
          }
          frame "Sequence: Switch" {
            # "#todo: add abort public method"
            # "#todo: make these separate states\n1. check B = Target?\n2. Turn on switch\n3. set PSU to target\n4. check hold OR psu = target\n5. set persist mode"
            n132 = Unbundle By Name(w384) -> ("Running Step"=w386:i32, "Self Reference"=w375:refnum<class "Instrument.OxfordVRM.lvclass">)
            n133 = case shown="\"Off\", Default" w378 {
              tunnel: [T5 "OFF" ("Switch Heater") T5 "ON" ("Switch Heater")] -> w382
              frame "Off", Default {
              }
              frame "On" {
              }
            }
            n134 = call "Set Switch Heater.vi"("error in (no error)"=w374, "Switch Heater"=w382, "Instrument.1820 in"=w375) -> ("error out"=w381:errorcluster)  [unwired: 6 in, 2 out]
            n135 = Increment(x=w386) -> (x+1=w385:i32)
            n136 = Bundle By Name(cluster=w384, "Running Step"=w385) -> (w383:T6)
            n137 = Format Into String(format string="%s >> %s", w379, w378) -> (resulting string=w373:string)  [unwired: 2 in, 1 out]
            n138 = call <vilib>:"Build State String with Arguments__JKI_lib_State_Machine.vi"("Arguments (\"\")"=w373, "State"="Sequence: Update Status") -> ("State with Arguments"=w376:string)  [unwired: 4 in]
            n139 = call <vilib>:"Add State(s) to Queue__jki_lib_state_machine.vi"("State(s) in Front (\"\")"=w376, "State(s) in (\"\")"=w389) -> ("States Out"=w388:string)  [unwired: 13 in]
          }
          frame "Sequence: Wait" {
            # "F = repeat this state. wait\nT = go to next state. don't wait"
            n140 = Unbundle By Name(w393) -> ("Running Step"=w416:i32)
            n141 = Equal?(x=w408, y="RESET") -> (x = y?=w412:bool)
            n142 = case shown="False" w412 {
              tunnel: [w422 u32 10000 ("time (ms)")] -> w411
              tunnel: [w425 w427] -> w398
              tunnel: w396 -> [w424 w427]
              tunnel: w408 -> [w423 _]
              frame False {
                n143 = Scan From String(format string="%d", input string=w423, error in=w424) -> (error out=w425:errorcluster, output 1=w421:i32)  [unwired: 2 in, 2 out]
                n144 = To Unsigned Long Integer(number=w421) -> (unsigned 32bit integer=w422:u32)
              }
              frame True {
              }
            }
            n145 = call <userlib>:"Periodic Trigger__ogtk.vi"("time (ms)"=w411, "reset"=w412) -> ("Triggered"=w413:bool, "timer value"=w410:u32)  [unwired: 11 in, 1 out]
            n146 = Or(x=w413, y=w412) -> (x .or. y?=w395:bool)
            n147 = Increment(x=w416) -> (x+1=w415:i32)
            n148 = Subtract(x=w411, y=w410) -> (x-y=w402:u32)
            "timer" <- w402
            n149 = Select(t=u32 0, s=w395, f=u32 100 ("milliseconds to wait")) -> (s? t:f=w400:u32)
            n150 = Select(t=w415, s=w395, f=w416) -> (s? t:f=w414:i32)
            n151 = call <userlib>:"Wait (ms)__ogtk.vi"("error in (no error)"=w398, "milliseconds to wait"=w400) -> ("error out"=w397:errorcluster)  [unwired: 8 in, 1 out]
            n152 = Bundle By Name(cluster=w393, "Running Step"=w414) -> (w417:T6)
            n153 = Divide(x=w402, y=u32 1000) -> (x/y=w404:dbl)
            n154 = Format Into String(format string="%s >> %d s", w407, w404) -> (resulting string=w405:string)  [unwired: 2 in, 1 out]
            n155 = call <vilib>:"Build State String with Arguments__JKI_lib_State_Machine.vi"("Arguments (\"\")"=w405, "State"="Sequence: Update Status") -> ("State with Arguments"=w392:string)  [unwired: 4 in]
            n156 = call <vilib>:"Add State(s) to Queue__jki_lib_state_machine.vi"("State(s) in Front (\"\")"=w392, "State(s) in (\"\")"=w420) -> ("States Out"=w419:string)  [unwired: 13 in]
          }
          frame "Sequence: Ramp PSU to Target" {
            # "#todo: add abort public method"
            # "#todo: make these separate states\n1. check B = Target?\n2. Turn on switch\n3. set PSU to target\n4. check hold OR psu = target\n5. set persist mode"
            n157 = Unbundle By Name(w440) -> ("Running Step"=w438:i32, "Self Reference"=w430:refnum<class "Instrument.OxfordVRM.lvclass">, "Field (T)"=w435:dbl, "Field Rate (T/min)"=w436:dbl)
            n158 = Increment(x=w438) -> (x+1=w437:i32)
            n159 = call "Get PSU Field.vi"("error in (no error)"=w429, "Instrument.1820 in"=w430) -> ("error out"=w441:errorcluster, "PSU Field (T)"=w443:dbl, "Instrument.1820 in"=w442:refnum<class "Instrument.OxfordVRM.lvclass">)  [unwired: 7 in]
            n160 = call "Instrument.1820.FloatApprox.vi"("y"=w435, "x"=w443) -> ("x ~ y?"=w444:bool)  [unwired: 4 in]
            n161 = case shown="False" w444 {
              tunnel: [w448 w457] -> _
              tunnel: [w450 w456] -> w434
              tunnel: w442 -> [w453 w457]
              tunnel: w441 -> [w452 w456]
              tunnel: w435 -> [w455 _]
              tunnel: w436 -> [w454 _]
              frame False {
                n162 = call "Set Target.vi"("error in (no error)"=w452, "Target Rate (T/min)"=w454, "Target Field (T)"=w455, "Instrument.1820 in"=w453) -> ("error out"=w451:errorcluster, "Instrument.1820 in"=w449:refnum<class "Instrument.OxfordVRM.lvclass">)  [unwired: 5 in, 1 out]
                n163 = call "Ramp to Set.vi"("error in (no error)"=w451, "Instrument.1820 in"=w449) -> ("error out"=w450:errorcluster, "Instrument.1820 in"=w448:refnum<class "Instrument.OxfordVRM.lvclass">)  [unwired: 7 in, 1 out]
              }
              frame True {
                # "If PSU Field == Target, do nothing"
              }
            }
            n164 = Bundle By Name(cluster=w440, "Running Step"=w437) -> (w439:T6)
            n165 = call <vilib>:"Build State String with Arguments__JKI_lib_State_Machine.vi"("Arguments (\"\")"=w431, "State"="Sequence: Update Status") -> ("State with Arguments"=w432:string)  [unwired: 4 in]
            n166 = call <vilib>:"Add State(s) to Queue__jki_lib_state_machine.vi"("State(s) in Front (\"\")"=w432, "State(s) in (\"\")"=w447) -> ("States Out"=w446:string)  [unwired: 13 in]
          }
          frame "Sequence: Ramp PSU to Magnet" {
            # "#todo: add abort public method"
            # "#todo: make these separate states\n1. check B = Target?\n2. Turn on switch\n3. set PSU to target\n4. check hold OR psu = target\n5. set persist mode"
            n167 = Unbundle By Name(w473) -> ("Running Step"=w471:i32, "Self Reference"=w459:refnum<class "Instrument.OxfordVRM.lvclass">)  [unwired: 2 out]
            n168 = call "Get PSU Field.vi"("error in (no error)"=w458, "Instrument.1820 in"=w459) -> ("error out"=w463:errorcluster, "PSU Field (T)"=w464:dbl, "Instrument.1820 in"=w465:refnum<class "Instrument.OxfordVRM.lvclass">)  [unwired: 7 in]
            n169 = Increment(x=w471) -> (x+1=w470:i32)
            n170 = call "Get Field.vi"("error in (no error)"=w463, "Instrument.1820 in"=w465) -> ("error out"=w467:errorcluster, "Field (T)"=w466:dbl, "Instrument.1820 in"=w468:refnum<class "Instrument.OxfordVRM.lvclass">)  [unwired: 7 in]
            n171 = call "Instrument.1820.FloatApprox.vi"("y"=w464, "x"=w466) -> ("x ~ y?"=w474:bool)  [unwired: 4 in]
            n172 = case shown="False" w474 {
              tunnel: [w480 w487] -> _
              tunnel: [w482 w486] -> w469
              tunnel: w468 -> [w485 w487]
              tunnel: w467 -> [w484 w486]
              tunnel: w466 -> [w479 _]
              frame False {
                n173 = call "Set Target.vi"("error in (no error)"=w484, "Target Rate (T/min)"=1.0, "Target Field (T)"=w479, "Instrument.1820 in"=w485) -> ("error out"=w483:errorcluster, "Instrument.1820 in"=w481:refnum<class "Instrument.OxfordVRM.lvclass">)  [unwired: 5 in, 1 out]
                n174 = call "Ramp to Set.vi"("error in (no error)"=w483, "Instrument.1820 in"=w481) -> ("error out"=w482:errorcluster, "Instrument.1820 in"=w480:refnum<class "Instrument.OxfordVRM.lvclass">)  [unwired: 7 in, 1 out]
              }
              frame True {
                # "If PSU Field == Magnet, do nothing"
              }
            }
            n175 = Bundle By Name(cluster=w473, "Running Step"=w470) -> (w472:T6)
            n176 = call <vilib>:"Build State String with Arguments__JKI_lib_State_Machine.vi"("Arguments (\"\")"=w460, "State"="Sequence: Update Status") -> ("State with Arguments"=w461:string)  [unwired: 4 in]
            n177 = call <vilib>:"Add State(s) to Queue__jki_lib_state_machine.vi"("State(s) in Front (\"\")"=w461, "State(s) in (\"\")"=w477) -> ("States Out"=w476:string)  [unwired: 13 in]
          }
          frame "Sequence: Ramp PSU to Zero" {
            # "#todo: add abort public method"
            # "#todo: make these separate states\n1. check B = Target?\n2. Turn on switch\n3. set PSU to target\n4. check hold OR psu = target\n5. set persist mode"
            n178 = Unbundle By Name(w497) -> ("Running Step"=w495:i32, "Self Reference"=w490:refnum<class "Instrument.OxfordVRM.lvclass">)
            n179 = call "Ramp to Zero.vi"("error in (no error)"=w489, "Instrument.1820 in"=w490) -> ("error out"=w488:errorcluster)  [unwired: 7 in, 2 out]
            n180 = Increment(x=w495) -> (x+1=w494:i32)
            n181 = Bundle By Name(cluster=w497, "Running Step"=w494) -> (w496:T6)
            n182 = call <vilib>:"Build State String with Arguments__JKI_lib_State_Machine.vi"("Arguments (\"\")"=w492, "State"="Sequence: Update Status") -> ("State with Arguments"=w491:string)  [unwired: 4 in]
            n183 = call <vilib>:"Add State(s) to Queue__jki_lib_state_machine.vi"("State(s) in Front (\"\")"=w491, "State(s) in (\"\")"=w500) -> ("States Out"=w499:string)  [unwired: 13 in]
          }
          frame "Sequence: Check Hold" {
            # "F = repeat this state. wait\nT = go to next state. don't wait"
            n184 = Unbundle By Name(w512) -> ("Running Step"=w514:i32, "Self Reference"=w508:refnum<class "Instrument.OxfordVRM.lvclass">)
            n185 = call "Get Status.vi"("Instrument.1820 in"=w508) -> ("error out"=w502:errorcluster, "Status"=w516:T10)  [unwired: 7 in, 2 out]
            n186 = Unbundle By Name(w516) -> ("Holding"=w503:bool)
            n187 = Increment(x=w514) -> (x+1=w515:i32)
            n188 = Select(t=w515, s=w503, f=w514) -> (s? t:f=w513:i32)
            n189 = Select(t=u32 0, s=w503, f=u32 500 ("milliseconds to wait")) -> (s? t:f=w505:u32)
            n190 = Bundle By Name(cluster=w512, "Running Step"=w513) -> (w511:T6)
            n191 = call <userlib>:"Wait (ms)__ogtk.vi"("error in (no error)"=w502, "milliseconds to wait"=w505) -> ("error out"=w501:errorcluster)  [unwired: 8 in, 1 out]
            n192 = call <vilib>:"Build State String with Arguments__JKI_lib_State_Machine.vi"("Arguments (\"\")"=w509, "State"="Sequence: Update Status") -> ("State with Arguments"=w507:string)  [unwired: 4 in]
            n193 = call <vilib>:"Add State(s) to Queue__jki_lib_state_machine.vi"("State(s) in Front (\"\")"=w507, "State(s) in (\"\")"=w519) -> ("States Out"=w518:string)  [unwired: 13 in]
          }
          frame "Sequence: Check RTOS" {
            # "F = repeat this state. wait\nT = go to next state. don't wait"
            n194 = Unbundle By Name(w532) -> ("Running Step"=w534:i32, "Self Reference"=w528:refnum<class "Instrument.OxfordVRM.lvclass">)
            n195 = call "Get Status.vi"("error in (no error)"=w520, "Instrument.1820 in"=w528) -> ("error out"=w522:errorcluster, "Status"=w536:T10)  [unwired: 6 in, 2 out]
            n196 = Unbundle By Name(w536) -> ("Ramp to Setpoint"=w523:bool)
            n197 = Increment(x=w534) -> (x+1=w535:i32)
            n198 = Select(t=w535, s=w523, f=w534) -> (s? t:f=w533:i32)
            n199 = Select(t=u32 0, s=w523, f=u32 500 ("milliseconds to wait")) -> (s? t:f=w525:u32)
            n200 = Bundle By Name(cluster=w532, "Running Step"=w533) -> (w531:T6)
            n201 = call <userlib>:"Wait (ms)__ogtk.vi"("error in (no error)"=w522, "milliseconds to wait"=w525) -> ("error out"=w521:errorcluster)  [unwired: 8 in, 1 out]
            n202 = call <vilib>:"Build State String with Arguments__JKI_lib_State_Machine.vi"("Arguments (\"\")"=w529, "State"="Sequence: Update Status") -> ("State with Arguments"=w527:string)  [unwired: 4 in]
            n203 = call <vilib>:"Add State(s) to Queue__jki_lib_state_machine.vi"("State(s) in Front (\"\")"=w527, "State(s) in (\"\")"=w539) -> ("States Out"=w538:string)  [unwired: 13 in]
          }
          frame "Sequence: Check RTOZ" {
            # "F = repeat this state. wait\nT = go to next state. don't wait"
            n204 = Unbundle By Name(w552) -> ("Running Step"=w554:i32, "Self Reference"=w548:refnum<class "Instrument.OxfordVRM.lvclass">)
            n205 = call "Get Status.vi"("error in (no error)"=w540, "Instrument.1820 in"=w548) -> ("error out"=w542:errorcluster, "Status"=w556:T10)  [unwired: 6 in, 2 out]
            n206 = Unbundle By Name(w556) -> ("Ramp to Zero"=w543:bool)
            n207 = Increment(x=w554) -> (x+1=w555:i32)
            n208 = Select(t=w555, s=w543, f=w554) -> (s? t:f=w553:i32)
            n209 = Bundle By Name(cluster=w552, "Running Step"=w553) -> (w551:T6)
            n210 = Select(t=u32 0, s=w543, f=u32 500 ("milliseconds to wait")) -> (s? t:f=w545:u32)
            n211 = call <userlib>:"Wait (ms)__ogtk.vi"("error in (no error)"=w542, "milliseconds to wait"=w545) -> ("error out"=w541:errorcluster)  [unwired: 8 in, 1 out]
            n212 = call <vilib>:"Build State String with Arguments__JKI_lib_State_Machine.vi"("Arguments (\"\")"=w549, "State"="Sequence: Update Status") -> ("State with Arguments"=w547:string)  [unwired: 4 in]
            n213 = call <vilib>:"Add State(s) to Queue__jki_lib_state_machine.vi"("State(s) in Front (\"\")"=w547, "State(s) in (\"\")"=w559) -> ("States Out"=w558:string)  [unwired: 13 in]
          }
          frame "Sequence: Check PSU at Zero" {
            # "F = repeat this state. wait\nT = go to next state. don't wait"
            n214 = Unbundle By Name(w577) -> ("Running Step"=w572:i32, "Self Reference"=w567:refnum<class "Instrument.OxfordVRM.lvclass">)
            n215 = call "Get PSU Field.vi"("error in (no error)"=w562, "Instrument.1820 in"=w567) -> ("error out"=w561:errorcluster, "PSU Field (T)"=w575:dbl)  [unwired: 7 in, 1 out]
            n216 = call "Instrument.1820.FloatApprox.vi"("y"=0.0, "x"=w575) -> ("x ~ y?"=w563:bool)  [unwired: 4 in]
            n217 = Increment(x=w572) -> (x+1=w573:i32)
            n218 = Select(t=w573, s=w563, f=w572) -> (s? t:f=w571:i32)
            n219 = Bundle By Name(cluster=w577, "Running Step"=w571) -> (w576:T6)
            n220 = Select(t=u32 0, s=w563, f=u32 500 ("milliseconds to wait")) -> (s? t:f=w565:u32)
            n221 = call <userlib>:"Wait (ms)__ogtk.vi"("error in (no error)"=w561, "milliseconds to wait"=w565) -> ("error out"=w560:errorcluster)  [unwired: 8 in, 1 out]
            n222 = call <vilib>:"Build State String with Arguments__JKI_lib_State_Machine.vi"("Arguments (\"\")"=w568, "State"="Sequence: Update Status") -> ("State with Arguments"=w569:string)  [unwired: 4 in]
            n223 = call <vilib>:"Add State(s) to Queue__jki_lib_state_machine.vi"("State(s) in Front (\"\")"=w569, "State(s) in (\"\")"=w580) -> ("States Out"=w579:string)  [unwired: 13 in]
          }
          frame "Sequence: Check Targets Match" {
            w583 = "" ("State")
            # "F = repeat this state. wait\nT = go to next state. don't wait"
            n224 = Unbundle By Name(w604) -> ("Running Step"=w601:i32, "Self Reference"=w593:refnum<class "Instrument.OxfordVRM.lvclass">, "Field (T)"=w589:dbl, "Field Rate (T/min)"=w587:dbl)
            n225 = call "Get Target.vi"("error in (no error)"=w592, "Instrument.1820 in"=w593) -> ("error out"=w591:errorcluster, "Target Field Rate (T/min)"=w588:dbl, "Target Field (T)"=w590:dbl)  [unwired: 6 in, 1 out]
            n226 = call "Instrument.1820.FloatApprox.vi"("y"=w589, "x"=w590) -> ("x ~ y?"=w586:bool)  [unwired: 4 in]
            n227 = call "Instrument.1820.FloatApprox.vi"("y"=w587, "x"=w588) -> ("x ~ y?"=w585:bool)  [unwired: 4 in]
            n228 = Increment(x=w601) -> (x+1=w602:i32)
            n229 = And(x=w586, y=w585) -> (x .and. y?=w584:bool)
            n230 = Select(t=w602, s=w584, f=w601) -> (s? t:f=w600:i32)
            n231 = Select(t=u32 0, s=w584, f=u32 500 ("milliseconds to wait")) -> (s? t:f=w595:u32)
            n232 = Select(t=w583, s=w584, f=w583) -> (s? t:f=w582:string)
            n233 = call <userlib>:"Wait (ms)__ogtk.vi"("error in (no error)"=w591, "milliseconds to wait"=w595) -> ("error out"=w597:errorcluster)  [unwired: 8 in, 1 out]
            n234 = Bundle By Name(cluster=w604, "Running Step"=w600) -> (w603:T6)
            n235 = call <vilib>:"Build State String with Arguments__JKI_lib_State_Machine.vi"("Arguments (\"\")"=w582, "State"=w582) -> ()  [unwired: 4 in, 1 out]
            n236 = call <vilib>:"Build State String with Arguments__JKI_lib_State_Machine.vi"("Arguments (\"\")"=w598, "State"="Sequence: Update Status") -> ("State with Arguments"=w581:string)  [unwired: 4 in]
            n237 = call <vilib>:"Add State(s) to Queue__jki_lib_state_machine.vi"("State(s) in Front (\"\")"=w581, "State(s) in (\"\")"=w607) -> ("States Out"=w606:string)  [unwired: 13 in]
          }
        }
      }
    }
    frame Error {
    }
  }
  n238 = call-parent "Process.vi"("error in"=w7, "Instrument"=w6) -> ("error out"=w4:errorcluster, "Instrument out"=→"Instrument.Example out":refnum<class "Instrument.OxfordVRM.lvclass">)  [unwired: 8 in]
  n239 = Merge Errors(w4, w3) -> (→"error out":errorcluster)
